vi "Protocol Engine.vi"(8 "error in (no error)":errorcluster, 10 "Parameters":T1 {"Compiled"."MetaData"."Refs"."Data Reference" format="%.0x"; "Compiled"."Triggers"."Chan Refs" format="%.0x"; "Compiled"."Statuses"."Refs" format="%.0x"; "Compiled"."Data"."Refs" format="%.0x"; "Compiled"."Periodic Enable"."Refs"."Data Reference" format="%.0x"; "Compiled"."Wait Values"."Refs"."Data Reference" format="%.0x"; "Compiled"."External Channels"."Channels" format="%.0x"; "Compiled"."External Channels"."Triggers" format="%.0x"}, 11 "State Variables":T14) -> (0 "error out":errorcluster)   [LabVIEW 2015, in "Instrument Addon Engine.lvlib"]
uses:
  Instrument Addon Engine.lvlib
  Inline Async API/Controls/Engine State Variables.ctl
  Network Communication/TCP Refs.ctl
  Network Communication/Network Comm Global Ref.ctl
  Stop FG/Stop Global Ref.ctl
  <vilib>/NI/AMC/Message Queue.ctl
  <vilib>/NI/AMC/Message.ctl
  <vilib>/NI/Tools/Keyed Array/KeyedArray.ctl
  Types/Commands RT Configuration Cluster.ctl
  Protocols.lvlibp/Protocol Parent/Protocol Parent.lvclass
  Shared/Types/Compiled Settings.ctl
  Shared/Types/Command Parameters.ctl
  Shared/Types/Linked Channel Cluster.ctl
  <vilib>/NI Veristand/Custom Device API/Block Data Reference.ctl
  <vilib>/NI Veristand/Custom Device API/Data Reference.ctl
  Shared/Types/Response RT Configuration Cluster.ctl
  Shared/Types/Response Parameters.ctl
  Shared/Types/Response Wait Type.ctl
  Shared/Types/Message Parameters.ctl
  Shared/Types/Message Generation Type.ctl
  Shared/Types/External Trigger Refs.ctl
  Types/FIFO References.ctl
  Protections.lvlibp/Parent Protection/Protection.lvclass
  Stop FG/Stop Global Commands.ctl
  Types/Buffered RT Instrument Command.ctl
  Protocols.lvlibp/Protocol Parent/Methods/Read Parameter.ctl
  Types/Buffered RT Instrument Request.ctl
  <vilib>/NI/AMC/Read Termination Message.vi
  <vilib>/NI/AMC/Create Single Message.vi
  <vilib>/NI/AMC/Update Message Routing Info.vi
  <vilib>/NI/Tools/Keyed Array/Map String.vi
  <vilib>/NI/Tools/String/Get Case Matching.vi
  <vilib>/NI/AMC/Send Message.vi
  Shared/Constants.vi
  <vilib>/NI/AMC/Globals.vi
  Stop FG/Stop FG.lvlib
  Error Handling API/Error Handling API.lvlib
  <vilib>/NI/AMC/AMC.lvlib
  <vilib>/NI/Tools/Keyed Array/Tools_KeyedArray.lvlib
  Shared/Instrument Addon Shared.lvlib
  Network Communication/Network Common API.lvlib
  Inline Async API/Inline Async API.lvlib
  <vilib>/NI Veristand/Custom Device API/Custom Device API.lvlib
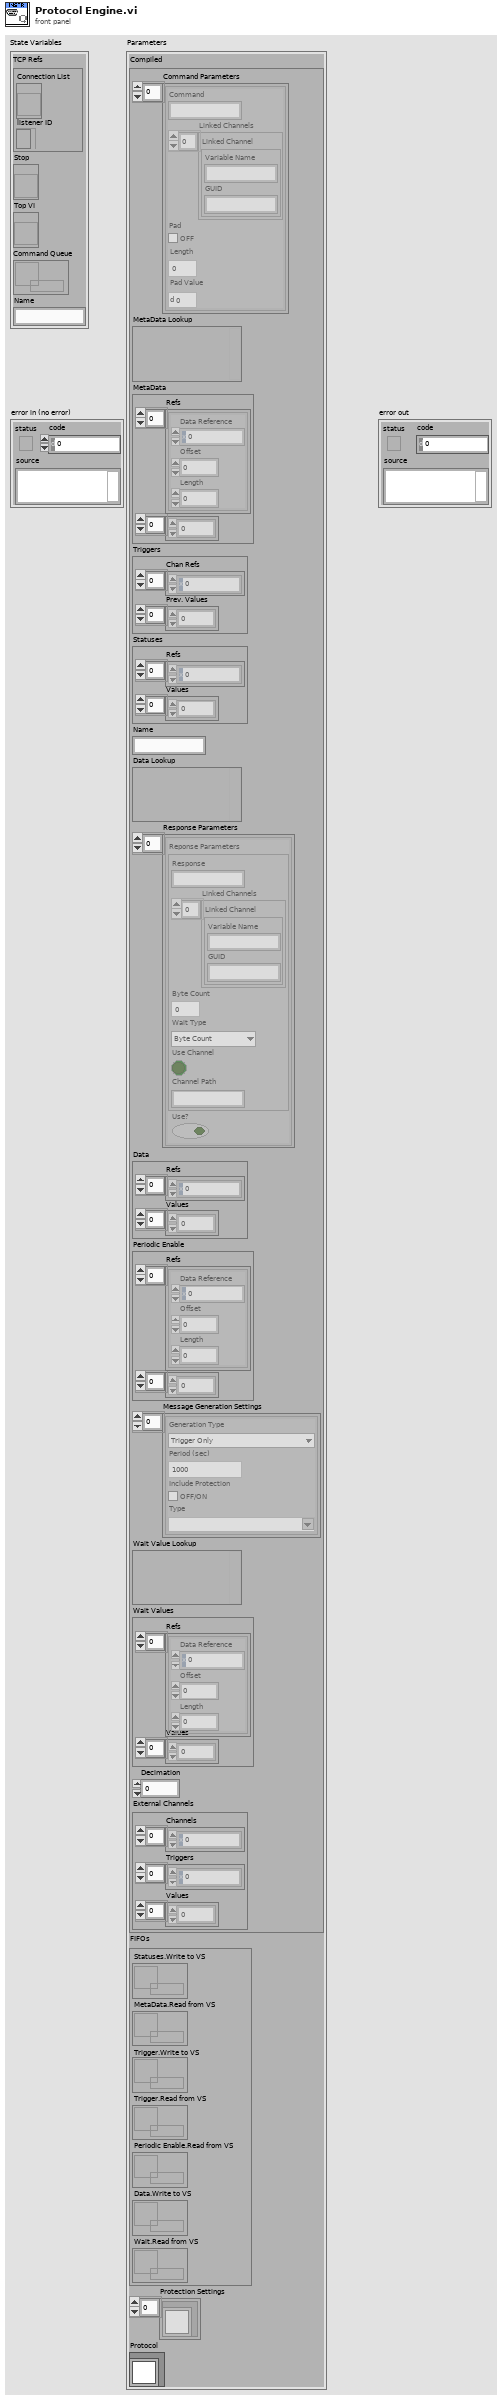
[diagram p1: front panel]
types:
  T1 = typedef "Instrument Addon Engine.lvlib/Commands RT Configuration Cluster.ctl" = cluster{"Compiled":T2, "FIFOs":T13, "Protection Settings":refnum<class "Protection.lvclass">[], "Protocol":refnum<class "Protocol Parent.lvclass">}
  T2 = typedef "Instrument Addon Shared.lvlib/Compiled Settings.ctl" = cluster{"Command Parameters":T3[], "MetaData Lookup":variant, "MetaData":cluster{"Refs":T5[], "Values":dbl[]}, "Triggers":cluster{"Chan Refs":T6[], "Prev. Values":dbl[]}, "Statuses":cluster{"Refs":T6[], "Values":dbl[]}, "Name":string, "Data Lookup":variant, "Response Parameters":T7[], "Data":cluster{"Refs":T6[], "Values":dbl[]}, "Periodic Enable":cluster{"Refs":T5[], "Values":dbl[]}, "Message Generation Settings":T10[], "Wait Value Lookup":variant, "Wait Values":cluster{"Refs":T5[], "Values":dbl[]}, "Decimation":u32, "External Channels":T12}
  T3 = typedef "Instrument Addon Shared.lvlib/Command Parameters.ctl" = cluster{"Command":string, "Linked Channels":T4[], "Pad":bool, "Length":u32, "Pad Value":u8}
  T4 = typedef "Instrument Addon Shared.lvlib/Linked Channel Cluster.ctl" = cluster{"Variable Name":string, "GUID":string}
  T5 = typedef "Custom Device API.lvlib/Block Data Reference.ctl" = cluster{"Data Reference":T6, "Offset":u64, "Length":u64}
  T6 = typedef "Custom Device API.lvlib/Data Reference.ctl" = i32
  T7 = typedef "Instrument Addon Shared.lvlib/Response RT Configuration Cluster.ctl" = cluster{"Reponse Parameters":T8, "Use?":bool}
  T8 = typedef "Instrument Addon Shared.lvlib/Response Parameters.ctl" = cluster{"Response":string, "Linked Channels":T4[], "Type Value":dbl, "Wait Type":T9, "Use Channel":bool, "Channel Path":string}
  T9 = typedef "Instrument Addon Shared.lvlib/Response Wait Type.ctl" = enum16{"Byte Count", "Wait sec"}
  T10 = typedef "Instrument Addon Shared.lvlib/Message Parameters.ctl" = cluster{"Generation Type":T11, "Period":dbl, "Include Protection":bool, "Type":string}
  T11 = typedef "Instrument Addon Shared.lvlib/Message Generation Type.ctl" = enum16{"Trigger Only", "Periodic & Trigger"}
  T12 = typedef "Instrument Addon Shared.lvlib/External Trigger Refs.ctl" = cluster{"Channels":T6[], "Triggers":T6[], "Values":dbl[]}
  T13 = typedef "Instrument Addon Engine.lvlib/FIFO References.ctl" = cluster{"Statuses.Write to VS":refnum<k33>, "MetaData.Read from VS":refnum<k33>, "Trigger.Write to VS":refnum<k33>, "Trigger.Read from VS":refnum<k33>, "Periodic Enable.Read from VS":refnum<k33>, "Data.Write to VS":refnum<k33>, "Wait.Read from VS":refnum<k33>}
  T14 = typedef "Instrument Addon Engine.lvlib/Inline Async API.lvlib/Engine State Variables.ctl" = cluster{"TCP Refs":T15, "Stop":T17, "Top VI":refnum<vi>, "Command Queue":T18, "Name":string}
  T15 = typedef "Instrument Addon Engine.lvlib/Network Common API.lvlib/TCP Refs.ctl" = cluster{"Connection List":T16, "listener ID":refnum<k5>}
  T16 = typedef "Instrument Addon Engine.lvlib/Network Common API.lvlib/Network Comm Global Ref.ctl" = refnum<vi>
  T17 = typedef "Instrument Addon Engine.lvlib/Stop FG.lvlib/Stop Global Ref.ctl" = refnum<vi>
  T18 = typedef "AMC.lvlib/Message Queue.ctl" = refnum<queue>
  T19 = typedef "Instrument Addon Engine.lvlib/Stop FG.lvlib/Stop Global Commands.ctl" = enum16{"Write", "Read", "Reset"}
  T20 = typedef "Instrument Addon Engine.lvlib/Buffered RT Instrument Command.ctl" = cluster{"Command":string, "Response Expected?":bool, "Wait Type":T9, "Wait Value":dbl}
  T21 = typedef "Instrument Addon Engine.lvlib/Buffered RT Instrument Request.ctl" = cluster{"Response":string, "Error":errorcluster}
  T22 = typedef "Protocols.lvlibp/Protocol Parent.lvclass/Read Parameter.ctl" = cluster{"Wait Type":enum16{"Byte Count", "Wait sec"}, "Wait Value":dbl}
  T23 = typedef "AMC.lvlib/Message.ctl" = cluster{"name":string, "value":string, "attributes":T24, "receiver host":string, "receiver process":string, "source host":string, "source process":string, "priority message":bool, "acknowledge message":bool}
  T24 = typedef "Tools_KeyedArray.lvlib/KeyedArray.ctl" = cluster{"keys":string[], "values":string[]}
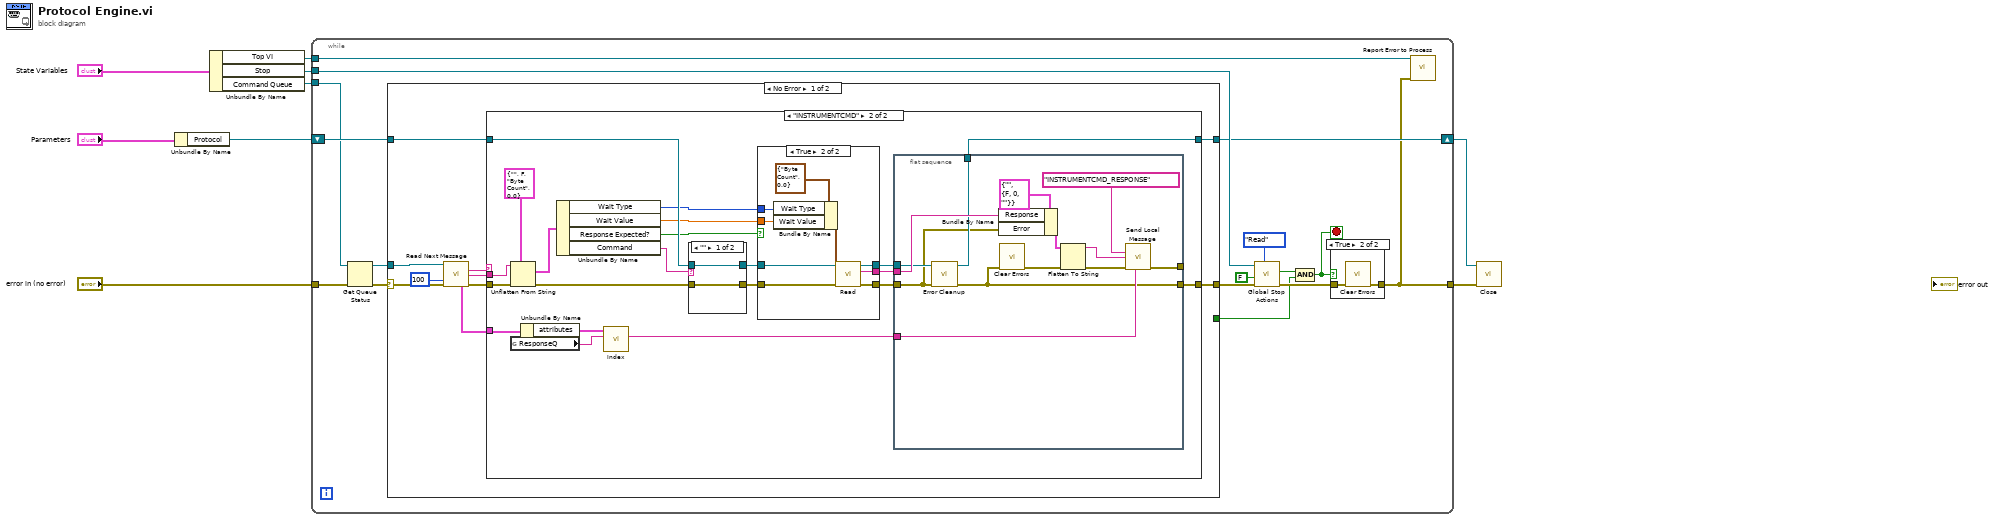
[diagram p0: block diagram]
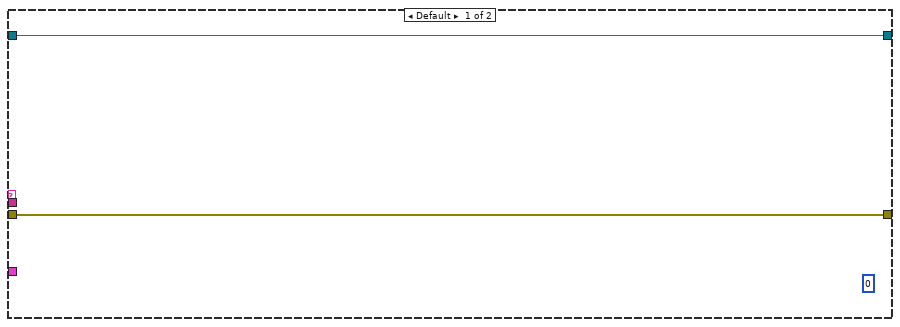
[diagram p2: hidden frame]
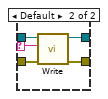
[diagram p3: hidden frame]
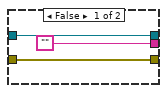
[diagram p4: hidden frame]
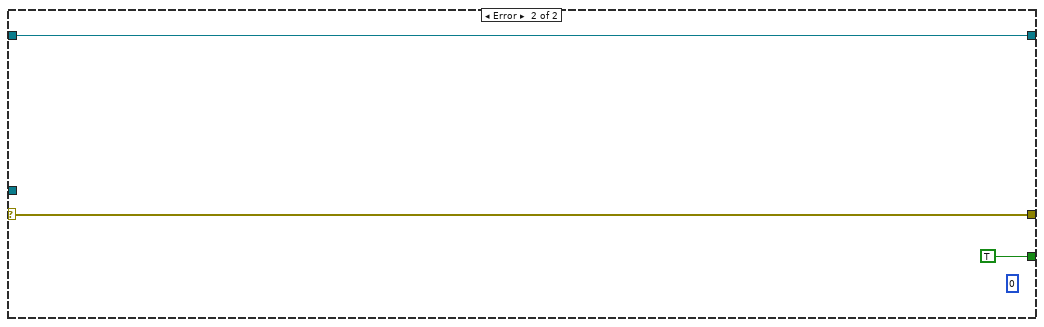
[diagram p5: hidden frame]
diagram:
  n1 = Unbundle By Name("Parameters") -> ("Protocol"=w4:refnum<class "Protocol Parent.lvclass">)
  n2 = Unbundle By Name("State Variables") -> ("Top VI"=w3:refnum<vi>, "Stop"=w9:T17, "Command Queue"=w6:T18)
  n3 = while {
    tunnel: "error in (no error)" -> [w14]
    tunnel: [w15] -> w1
    tunnel: w9 -> [w23]
    tunnel: w3 -> [w21]
    tunnel: w6 -> [w13]
    shift-right: [w18] -> w2
    shift-left: w4 -> [w19]
    stop <- w17 stop-if-true
    n4 = Get Queue Status(queue=w13, error in (no error)=w14) -> (queue out=w12:T18, error out=w10:errorcluster)  [unwired: 1 in, 6 out]
    n5 = case shown="No Error" w10 {
      selector: w10 -> [w26 w93]
      tunnel: [w31 w93] -> w20
      tunnel: w19 -> [w30 w92]
      tunnel: [w29 w92] -> w18
      tunnel: w12 -> [w27 _]
      tunnel: [_ TRUE] -> w11
      frame No Error {
        n6 = call <vilib>:"Read Next Message.vi"("message queue in"=w27, "timeout (1 ms)"=100, "error in"=w26) -> ("message name"=w33:string, "message value"=w34:string, "message"=w35:T23, "error out"=w28:errorcluster)  [unwired: 5 in, 4 out]
        n7 = case shown="\"INSTRUMENTCMD\"" w33 {
          tunnel: w28 -> [w37 w54]
          tunnel: w34 -> [_ w58]
          tunnel: w30 -> [w36 w56]
          tunnel: [w37 w47] -> w31
          tunnel: w35 -> [_ w46]
          tunnel: [w36 w38] -> w29
          frame Default {
            (unwired) u32 0
          }
          frame "INSTRUMENTCMD" {
            n8 = Unflatten From String(type=T20 {"Command"="", "Response Expected?"=FALSE, "Wait Type"=enum."Byte Count", "Wait Value"=0.0} ("Buffered Command Cluster"), binary string=w58, error in (no error)=w54) -> (value=w51:T20, error out=w53:errorcluster)  [unwired: 2 in, 1 out]
            n9 = global read "Constants.vi" "ResponseQ"() -> (w42:string)
            n10 = Unbundle By Name(w46) -> ("attributes"=w44:T24)
            n11 = Unbundle By Name(w51) -> ("Wait Type"=w45:T9, "Wait Value"=w41:dbl, "Response Expected?"=w50:bool, "Command"=w40:string)
            n12 = call <vilib>:"Index.vi"("key"=w42, "array in"=w44) -> ("value"=w43:string)  [unwired: 3 in, 2 out]
            n13 = case shown="\"\"" w40 {
              selector: w40 -> [_ w61]
              tunnel: [w59 w65] -> w57
              tunnel: w56 -> [w60 w64]
              tunnel: [w60 w63] -> w55
              tunnel: w53 -> [w59 w62]
              frame "" {
              }
              frame Default {
                n14 = call-dynamic "Write.vi"("error in (no error)"=w62, "String"=w61, "Protocol Parent in"=w64) -> ("error out"=w65:errorcluster, "Protocol Parent out"=w63:refnum<class "Protocol Parent.lvclass">)  [unwired: 7 in]
              }
            }
            n15 = case shown="True" w50 {
              tunnel: w57 -> [w81 w88]
              tunnel: w55 -> [w79 w87]
              tunnel: [w81 w90] -> w49
              tunnel: ["" w89] -> w48
              tunnel: w45 -> [_ w84]
              tunnel: w41 -> [_ w86]
              tunnel: [w79 w85] -> w39
              frame False {
              }
              frame True {
                n16 = Bundle By Name(cluster=T22 {"Wait Type"=enum."Byte Count", "Wait Value"=0.0} ("Read Parameter"), "Wait Type"=w84, "Wait Value"=w86) -> (w82:T22)
                n17 = call-dynamic "Read.vi"("error in (no error)"=w88, "Variant"=w82, "Protocol Parent in"=w87) -> ("error out"=w90:errorcluster, "String"=w89:string, "Protocol Parent out"=w85:refnum<class "Protocol Parent.lvclass">)  [unwired: 6 in]
              }
            }
            n18 = flat-sequence {
              tunnel: w49 -> [w66]
              tunnel: w48 -> [w77]
              tunnel: [w69] -> w47
              tunnel: [w71] -> _
              tunnel: w43 -> [w70]
              tunnel: w39 -> [w68]
              tunnel: [w67] -> w38
              frame #0 {
                n19 = call-dynamic "Error Cleanup.vi"("error in (no error)"=w66, "Protocol Parent in"=w68) -> ("error out"=w69:errorcluster, "Protocol Parent out"=w67:refnum<class "Protocol Parent.lvclass">)  [unwired: 8 in]
                n20 = Bundle By Name(cluster=T21 {"Response"="", "Error"={"status"=FALSE, "code"=0, "source"=""}}, "Response"=w77, "Error"=w66) -> (w76:T21)
                n21 = call <vilib>:"Clear Errors.vi"("error in (no error)"=w69) -> ("error out"=w75:errorcluster)  [unwired: 5 in, 1 out]
                n22 = Flatten To String(anything=w76, error in (no error)=w75) -> (data string=w73:string, error out=w74:errorcluster)  [unwired: 2 in, 1 out]
                n23 = call <vilib>:"Send Local Message.vi"("receiver process (\"\" - local)"=w70, "message name"="INSTRUMENTCMD_RESPONSE", "message value"=w73, "error in"=w74) -> ("error out"=w71:errorcluster)  [unwired: 9 in, 2 out]
              }
            }
          }
        }
      }
      frame Error {
        (unwired) u32 0
      }
    }
    n24 = call "Global Stop Actions.vi"("Command"=Stop_Global_Commands."Read", "error in (no error)"=w20, "Stop on Error?"=FALSE, "vi reference"=w23) -> ("error out"=w16:errorcluster, "Latched Stop"=w24:bool)  [unwired: 5 in, 1 out]
    n25 = Compound Arithmetic op=AND(w24, w11) -> (w17:bool)
    n26 = case shown="True" w17 {
      tunnel: w16 -> [w94 w96]
      tunnel: [w94 w95] -> w15
      frame False {
      }
      frame True {
        n27 = call <vilib>:"Clear Errors.vi"("error in (no error)"=w96) -> ("error out"=w95:errorcluster)  [unwired: 5 in, 1 out]
      }
    }
    n28 = call "Report Error to Process.vi"("Error"=w15, "This VI"=w21) -> ()  [unwired: 10 in]
  }
  n29 = call-dynamic "Close.vi"("error in (no error)"=w1, "Protocol Parent in"=w2) -> ()  [unwired: 8 in, 2 out]
